vi "move_5.vi"(6 "Array 4":i32[](array[numeric]), 9 "Array 6":i32[](array[numeric]), 10 "Array in":i32[](array[numeric]), 11 "Enum in":enum16{"move4", "move4_1", "move4_2"}(ring)) -> (1 "Array 3":i32[](array[numeric]), 2 "Array out":i32[](array[numeric]), 3 "Enum out":T1(ring), 4 "Array 5":i32[](array[numeric]))   [LabVIEW 2016]
uses:
  <vilib>/NXT/Block Support/NXT_OutputPort.ctl
  <vilib>/NXT/NXTIO Xnodes/NXTIONodeSubVIs/NXTStopMotors.vi
  <vilib>/NXT/NXTIO Xnodes/NXTIONodeSubVIs/NXTMotorRunDistance.vi
  <vilib>/NXT/NXTIO Xnodes/NXTIONodeSubVIs/LEGOMotorStatus.vi
  <vilib>/NXT/NXTIO Xnodes/NXTIONodeSubVIs/NXTMoveMotors.vi
  <vilib>/NXT/NXTIO Xnodes/NXTIONodeSubVIs/LEGOResetMotors.vi
  <vilib>/NXT/Subs/LVHSConnector.ctl
  <vilib>/NXT/NXTIO Xnodes/AddressXNode/NXTIOAddress.xnode
  <vilib>/NXT/NXTIO Xnodes/NXTIOXNode/NXTIO.xnode
  <vilib>/NXT/LegoClasses/BrickReference/BrickReference.lvclass
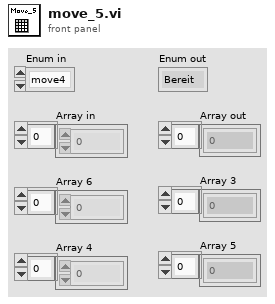
[diagram p1: front panel]
types:
  T1 = enum16{"Bereit", "Move 1", "Reference_pos", "Wait", "row1_check", "row2_check", "row3_check", "return", "move2", "move3", "move4", "move5", "end"}
  T2 = enum16{"forward", "right", "mark", "pause", "up", "return", "end"}
  T3 = typedef "NXT_OutputPort.ctl" = u8
  T4 = cluster{"Output Port":T3, "Output Port 2":T3, "Output Port 3":T3}
  T5 = enum16{"forward", "mark", "pause", "up", "return", "end"}
  T6 = typedef "LVHSConnector.ctl" = refnum<class "BrickReference.lvclass">
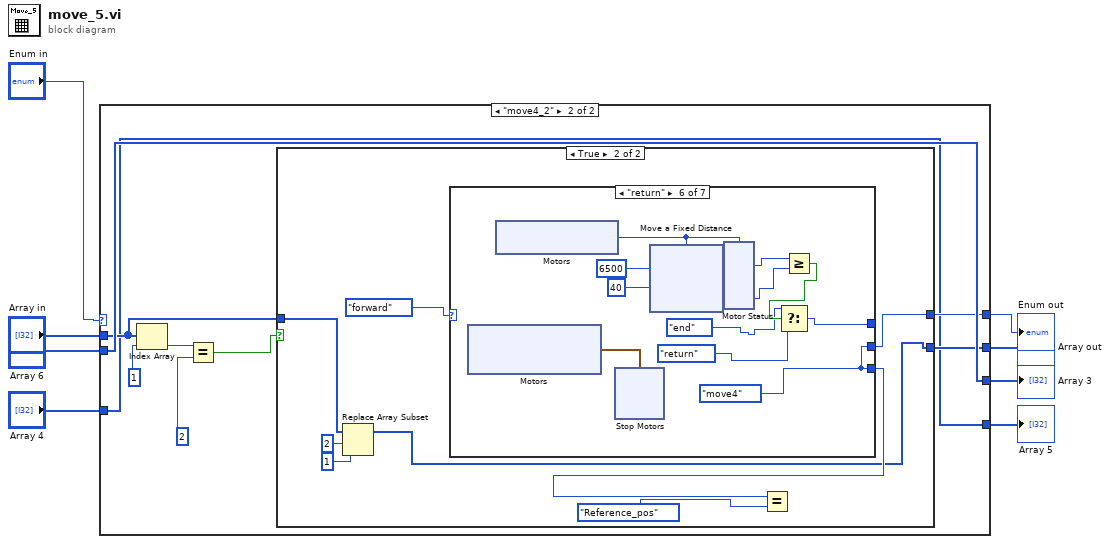
[diagram p0: block diagram]
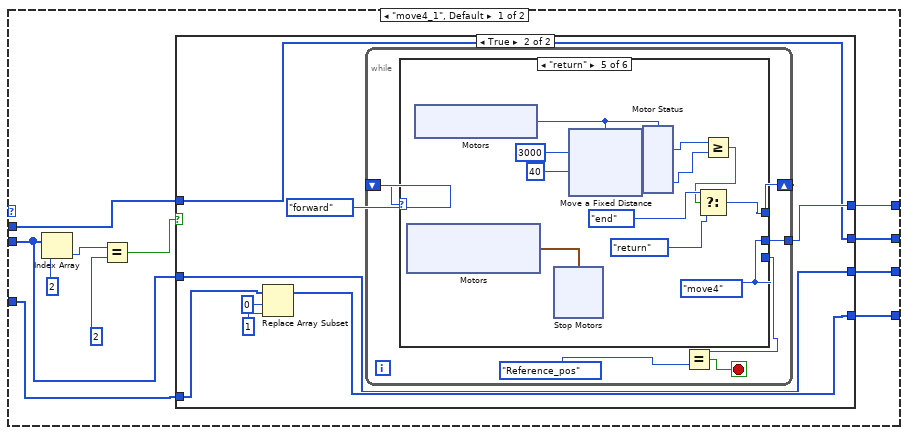
[diagram p2: hidden frame]
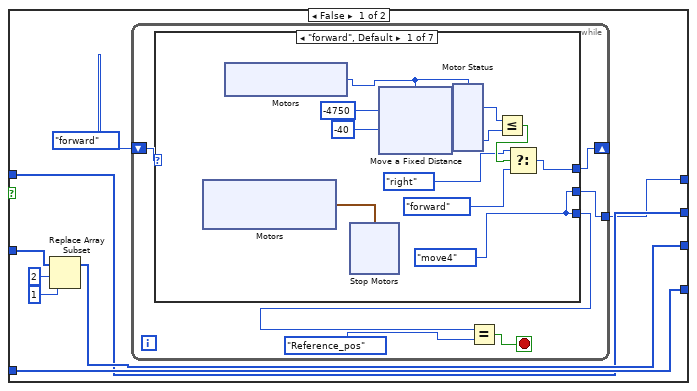
[diagram p3: hidden frame]
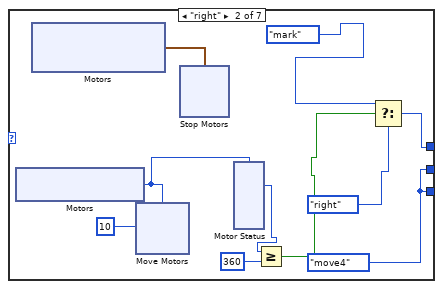
[diagram p4: hidden frame]
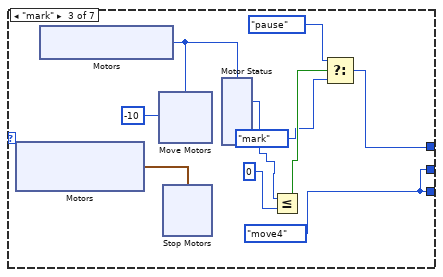
[diagram p5: hidden frame]
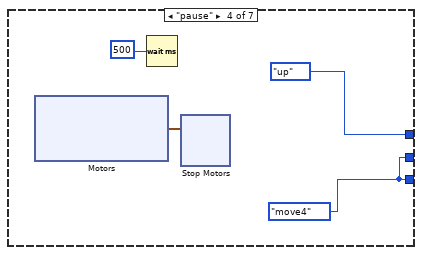
[diagram p6: hidden frame]
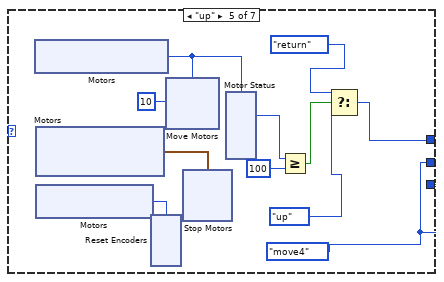
[diagram p7: hidden frame]
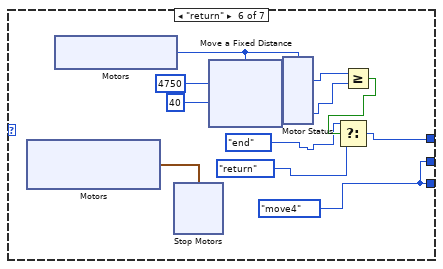
[diagram p8: hidden frame]
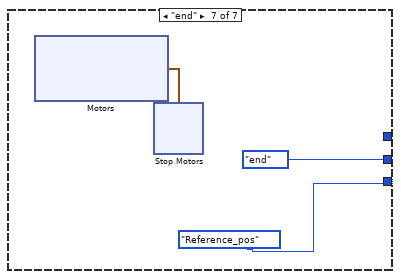
[diagram p9: hidden frame]
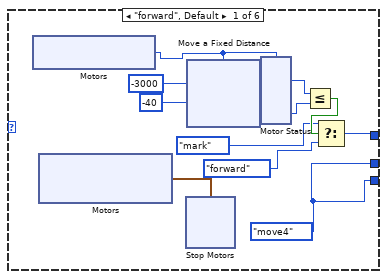
[diagram p10: hidden frame]
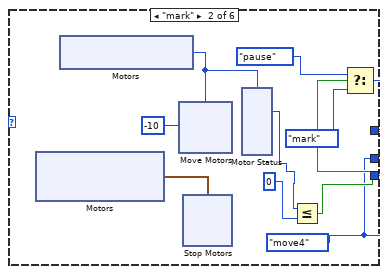
[diagram p11: hidden frame]
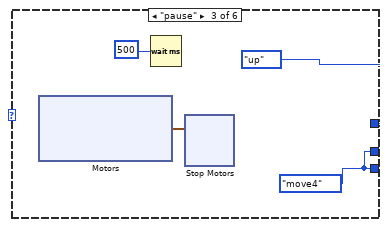
[diagram p12: hidden frame]
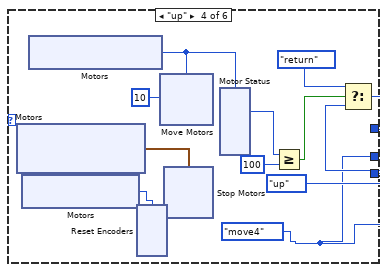
[diagram p13: hidden frame]
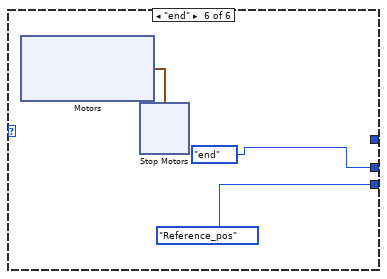
[diagram p14: hidden frame]
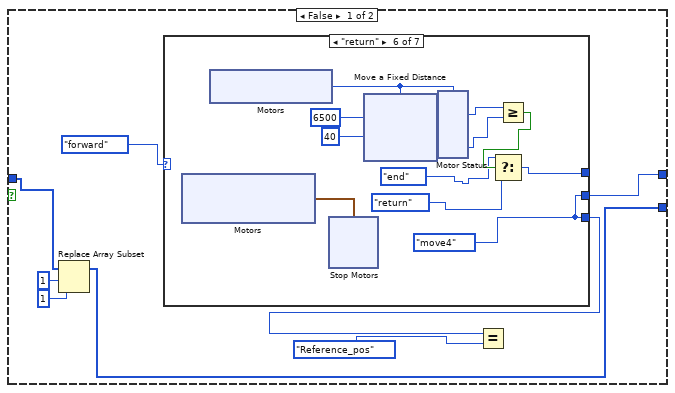
[diagram p15: hidden frame]
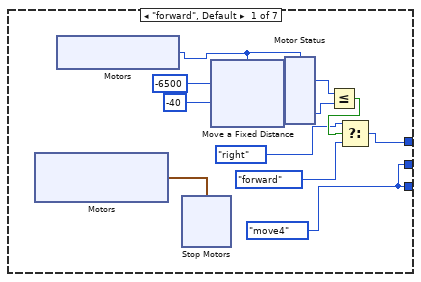
[diagram p16: hidden frame]
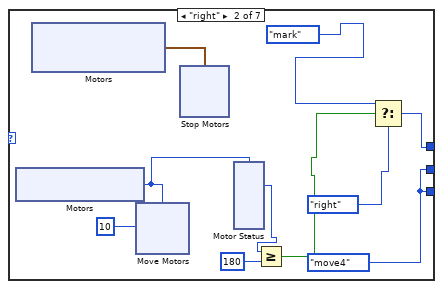
[diagram p17: hidden frame]
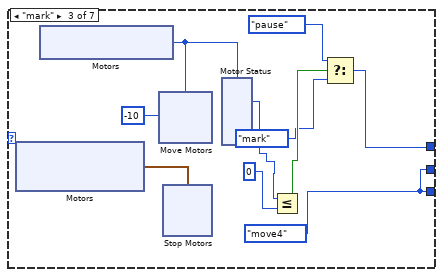
[diagram p18: hidden frame]
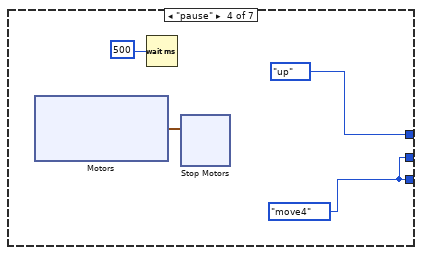
[diagram p19: hidden frame]
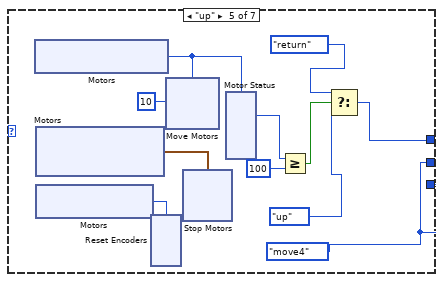
[diagram p20: hidden frame]
diagram:
  n1 = case shown="\"move4_2\"" "Enum in" {
    tunnel: "Array 6" -> [w13 w406]
    tunnel: [w15 w402] -> w2
    tunnel: "Array 4" -> [w14 w402]
    tunnel: [w12 w406] -> w4
    tunnel: [w11 w404] -> w5
    tunnel: "Array in" -> [w10 w405]
    tunnel: [w9 w403] -> w7
    frame "move4_1", Default {
      n2 = Index Array(array=w13, index=2) -> (element=w16:i32)
      n3 = Equal?(x=w16, y=2 ("element")) -> (x = y?=w18:bool)
      n4 = case shown="True" w18 {
        tunnel: [w24 w230] -> w15
        tunnel: w14 -> [w24 w231]
        tunnel: w13 -> [w23 w228]
        tunnel: [w22 w228] -> w12
        tunnel: [w21 w227] -> w11
        tunnel: w10 -> [w21 w227]
        tunnel: [w20 w229] -> w9
        frame False {
          n5 = Replace Array Subset(array=w23, new element=1 ("new element/subarray"), index=2) -> (w22:i32[])
          n6 = while {
            shift-right: [w29] -> _
            shift-left: T2."forward" -> [w30]
            tunnel: [w28] -> w20
            stop <- w32 stop-if-true
            n7 = case shown="\"forward\", Default" w30 {
              tunnel: [w34 w71 w103 T2."up" w146 w182 _] -> w29
              tunnel: [w43 w70 w102 w134 w145 w191 T1."Reference_pos"] -> w33
              tunnel: [w43 w70 w102 w134 w145 w191 T1."end"] -> w28
              frame "forward", Default {
                w39 = -4750 ("Distance 1")
                w43 = T1."move4"
                n8 = xnode "Motors"() -> ("Motor"=w44:cluster{"Port":T3, "Port":T3})
                n9 = xnode "Motors"() -> ("Motor"=w38:T3)
                n10 = xnode "Stop Motors"("Motors"=w44) -> ()  [unwired: 1 in, 1 out]
                n11 = xnode "Move a Fixed Distance"("Speed 1"=i8 -40, "Distance 1"=w39, "Motors"=w38) -> ("NXT/EV3"=w40:T6)  [unwired: 1 in]
                n12 = xnode "Motor Status"("Motors"=w38, "NXT/EV3"=w40) -> ("Position 1"=w41:i32)  [unwired: 2 out]
                n13 = Less Or Equal?(x=w41, y=w39) -> (x <= y?=w37:bool)
                n14 = Select(t=T2."right", s=w37, f=T2."forward") -> (s? t:f=w34:T2)
              }
              frame "right" {
                w70 = T1."move4"
                n15 = xnode "Motors"() -> ("Motor"=w79:T3)
                n16 = xnode "Motors"() -> ("Motor"=w78:cluster{"Port":T3, "Port":T3})
                n17 = xnode "Move Motors"("Power/Speed 1"=i8 10, "Motors"=w79) -> ()  [unwired: 1 in, 1 out]
                n18 = xnode "Stop Motors"("Motors"=w78) -> ()  [unwired: 1 in, 1 out]
                n19 = xnode "Motor Status"("Motors"=w79) -> ("Position 1"=w76:i32)  [unwired: 1 in, 2 out]
                n20 = Greater Or Equal?(x=w76, y=360) -> (x >= y?=w75:bool)
                n21 = Select(t=T2."mark", s=w75, f=T2."right") -> (s? t:f=w71:T2)
              }
              frame "mark" {
                w102 = T1."move4"
                n22 = xnode "Motors"() -> ("Motor"=w111:cluster{"Port":T3, "Port":T3})
                n23 = xnode "Motors"() -> ("Motor"=w109:T3)
                n24 = xnode "Move Motors"("Power/Speed 1"=i8 -10, "Motors"=w109) -> ()  [unwired: 1 in, 1 out]
                n25 = xnode "Stop Motors"("Motors"=w111) -> ()  [unwired: 1 in, 1 out]
                n26 = xnode "Motor Status"("Motors"=w109) -> ("Position 1"=w108:i32)  [unwired: 1 in, 2 out]
                n27 = Less Or Equal?(x=w108, y=0) -> (x <= y?=w106:bool)
                n28 = Select(t=T2."pause", s=w106, f=T2."mark") -> (s? t:f=w103:T2)
              }
              frame "pause" {
                w134 = T1."move4"
                n29 = xnode "Motors"() -> ("Motor"=w137:cluster{"Port":T3, "Port":T3, "Port":T3})
                n30 = Wait (ms)(milliseconds to wait=u32 500 ("millisecond timer value")) -> ()  [unwired: 1 out]
                n31 = xnode "Stop Motors"("Motors"=w137) -> ()  [unwired: 1 in, 1 out]
              }
              frame "up" {
                w145 = T1."move4"
                n32 = xnode "Motors"() -> ("Motor"=w150:T3)
                n33 = xnode "Motors"() -> ("Motor"=w153:cluster{"Port":T3, "Port":T3})
                n34 = xnode "Motors"() -> ("Motor"=w144:T3)
                n35 = xnode "Reset Encoders"("Motors"=w144) -> ()  [unwired: 1 in, 1 out]
                n36 = xnode "Move Motors"("Power/Speed 1"=i8 10, "Motors"=w150) -> ()  [unwired: 1 in, 1 out]
                n37 = xnode "Stop Motors"("Motors"=w153) -> ()  [unwired: 1 in, 1 out]
                n38 = xnode "Motor Status"("Motors"=w150) -> ("Position 1"=w151:i32)  [unwired: 1 in, 2 out]
                n39 = Greater Or Equal?(x=w151, y=100) -> (x >= y?=w152:bool)
                n40 = Select(t=T2."return", s=w152, f=T2."up") -> (s? t:f=w146:T2)
              }
              frame "return" {
                w186 = 4750 ("Distance 1")
                w191 = T1."move4"
                n41 = xnode "Motors"() -> ("Motor"=w192:cluster{"Port":T3, "Port":T3})
                n42 = xnode "Motors"() -> ("Motor"=w189:T3)
                n43 = xnode "Stop Motors"("Motors"=w192) -> ()  [unwired: 1 in, 1 out]
                n44 = xnode "Move a Fixed Distance"("Speed 1"=i8 40, "Distance 1"=w186, "Motors"=w189) -> ("NXT/EV3"=w188:T6)  [unwired: 1 in]
                n45 = xnode "Motor Status"("Motors"=w189, "NXT/EV3"=w188) -> ("Position 1"=w187:i32)  [unwired: 2 out]
                n46 = Greater Or Equal?(x=w187, y=w186) -> (x >= y?=w185:bool)
                n47 = Select(t=T2."end", s=w185, f=T2."return") -> (s? t:f=w182:T2)
              }
              frame "end" {
                n48 = xnode "Motors"() -> ("Motor"=w219:cluster{"Port":T3, "Port":T3, "Port":T3})
                n49 = xnode "Stop Motors"("Motors"=w219) -> ()  [unwired: 1 in, 1 out]
              }
            }
            n50 = Equal?(x=w33, y=T1."Reference_pos") -> (x = y?=w32:bool)
          }
        }
        frame True {
          n51 = Replace Array Subset(array=w231, new element=1 ("new element/subarray"), index=0) -> (w230:i32[])
          n52 = while {
            shift-right: [w240] -> _
            shift-left: T5."forward" -> [w239]
            tunnel: [w235] -> w229
            stop <- w237 stop-if-true
            n53 = case shown="\"return\"" w239 {
              tunnel: [w241 w284 T5."up" w326 w358 _] -> w240
              tunnel: [w250 w277 w309 w320 w366 T1."Reference_pos"] -> w238
              tunnel: [w250 w277 w309 w320 w366 T1."end"] -> w235
              frame "forward", Default {
                w246 = -3000 ("Distance 1")
                w250 = T1."move4"
                n54 = xnode "Motors"() -> ("Motor"=w245:T3)
                n55 = xnode "Motors"() -> ("Motor"=w251:cluster{"Port":T3, "Port":T3})
                n56 = xnode "Stop Motors"("Motors"=w251) -> ()  [unwired: 1 in, 1 out]
                n57 = xnode "Move a Fixed Distance"("Speed 1"=i8 -40, "Distance 1"=w246, "Motors"=w245) -> ("NXT/EV3"=w247:T6)  [unwired: 1 in]
                n58 = xnode "Motor Status"("Motors"=w245, "NXT/EV3"=w247) -> ("Position 1"=w248:i32)  [unwired: 2 out]
                n59 = Less Or Equal?(x=w248, y=w246) -> (x <= y?=w244:bool)
                n60 = Select(t=T5."mark", s=w244, f=T5."forward") -> (s? t:f=w241:T5)
              }
              frame "mark" {
                w277 = T1."move4"
                n61 = xnode "Motors"() -> ("Motor"=w286:cluster{"Port":T3, "Port":T3})
                n62 = xnode "Motors"() -> ("Motor"=w281:T3)
                n63 = xnode "Move Motors"("Power/Speed 1"=i8 -10, "Motors"=w281) -> ()  [unwired: 1 in, 1 out]
                n64 = xnode "Stop Motors"("Motors"=w286) -> ()  [unwired: 1 in, 1 out]
                n65 = xnode "Motor Status"("Motors"=w281) -> ("Position 1"=w280:i32)  [unwired: 1 in, 2 out]
                n66 = Less Or Equal?(x=w280, y=0) -> (x <= y?=w278:bool)
                n67 = Select(t=T5."pause", s=w278, f=T5."mark") -> (s? t:f=w284:T5)
              }
              frame "pause" {
                w309 = T1."move4"
                n68 = xnode "Motors"() -> ("Motor"=w312:cluster{"Port":T3, "Port":T3, "Port":T3})
                n69 = Wait (ms)(milliseconds to wait=u32 500 ("millisecond timer value")) -> ()  [unwired: 1 out]
                n70 = xnode "Stop Motors"("Motors"=w312) -> ()  [unwired: 1 in, 1 out]
              }
              frame "up" {
                w320 = T1."move4"
                n71 = xnode "Motors"() -> ("Motor"=w328:cluster{"Port":T3, "Port":T3})
                n72 = xnode "Motors"() -> ("Motor"=w319:T3)
                n73 = xnode "Motors"() -> ("Motor"=w322:T3)
                n74 = xnode "Reset Encoders"("Motors"=w319) -> ()  [unwired: 1 in, 1 out]
                n75 = xnode "Move Motors"("Power/Speed 1"=i8 10, "Motors"=w322) -> ()  [unwired: 1 in, 1 out]
                n76 = xnode "Stop Motors"("Motors"=w328) -> ()  [unwired: 1 in, 1 out]
                n77 = xnode "Motor Status"("Motors"=w322) -> ("Position 1"=w323:i32)  [unwired: 1 in, 2 out]
                n78 = Greater Or Equal?(x=w323, y=100) -> (x >= y?=w327:bool)
                n79 = Select(t=T5."return", s=w327, f=T5."up") -> (s? t:f=w326:T5)
              }
              frame "return" {
                w361 = 3000 ("Distance 1")
                w366 = T1."move4"
                n80 = xnode "Motors"() -> ("Motor"=w367:cluster{"Port":T3, "Port":T3})
                n81 = xnode "Motors"() -> ("Motor"=w364:T3)
                n82 = xnode "Stop Motors"("Motors"=w367) -> ()  [unwired: 1 in, 1 out]
                n83 = xnode "Move a Fixed Distance"("Speed 1"=i8 40, "Distance 1"=w361, "Motors"=w364) -> ("NXT/EV3"=w363:T6)  [unwired: 1 in]
                n84 = xnode "Motor Status"("Motors"=w364, "NXT/EV3"=w363) -> ("Position 1"=w362:i32)  [unwired: 2 out]
                n85 = Greater Or Equal?(x=w362, y=w361) -> (x >= y?=w357:bool)
                n86 = Select(t=T5."end", s=w357, f=T5."return") -> (s? t:f=w358:T5)
              }
              frame "end" {
                n87 = xnode "Motors"() -> ("Motor"=w395:cluster{"Port":T3, "Port":T3, "Port":T3})
                n88 = xnode "Stop Motors"("Motors"=w395) -> ()  [unwired: 1 in, 1 out]
              }
            }
            n89 = Equal?(x=w238, y=T1."Reference_pos") -> (x = y?=w237:bool)
          }
        }
      }
    }
    frame "move4_2" {
      n90 = Index Array(array=w405, index=1) -> (element=w407:i32)
      n91 = Equal?(x=w407, y=2 ("element")) -> (x = y?=w409:bool)
      n92 = case shown="True" w409 {
        tunnel: w405 -> [w413 w614]
        tunnel: [w412 w613] -> w404
        tunnel: [w411 w612] -> w403
        frame False {
          n93 = Replace Array Subset(array=w413, new element=1 ("new element/subarray"), index=1) -> (w412:i32[])
          n94 = case shown="\"return\"" T2."forward" {
            tunnel: [w419 w456 w488 T2."up" w531 w567 _] -> _
            tunnel: [w428 w455 w487 w519 w530 w576 T1."Reference_pos"] -> w416
            tunnel: [w428 w455 w487 w519 w530 w576 T1."end"] -> w411
            frame "forward", Default {
              w424 = -6500 ("Distance 1")
              w428 = T1."move4"
              n95 = xnode "Motors"() -> ("Motor"=w429:cluster{"Port":T3, "Port":T3})
              n96 = xnode "Motors"() -> ("Motor"=w423:T3)
              n97 = xnode "Stop Motors"("Motors"=w429) -> ()  [unwired: 1 in, 1 out]
              n98 = xnode "Move a Fixed Distance"("Speed 1"=i8 -40, "Distance 1"=w424, "Motors"=w423) -> ("NXT/EV3"=w425:T6)  [unwired: 1 in]
              n99 = xnode "Motor Status"("Motors"=w423, "NXT/EV3"=w425) -> ("Position 1"=w426:i32)  [unwired: 2 out]
              n100 = Less Or Equal?(x=w426, y=w424) -> (x <= y?=w422:bool)
              n101 = Select(t=T2."right", s=w422, f=T2."forward") -> (s? t:f=w419:T2)
            }
            frame "right" {
              w455 = T1."move4"
              n102 = xnode "Motors"() -> ("Motor"=w464:T3)
              n103 = xnode "Motors"() -> ("Motor"=w463:cluster{"Port":T3, "Port":T3})
              n104 = xnode "Move Motors"("Power/Speed 1"=i8 10, "Motors"=w464) -> ()  [unwired: 1 in, 1 out]
              n105 = xnode "Stop Motors"("Motors"=w463) -> ()  [unwired: 1 in, 1 out]
              n106 = xnode "Motor Status"("Motors"=w464) -> ("Position 1"=w461:i32)  [unwired: 1 in, 2 out]
              n107 = Greater Or Equal?(x=w461, y=180) -> (x >= y?=w460:bool)
              n108 = Select(t=T2."mark", s=w460, f=T2."right") -> (s? t:f=w456:T2)
            }
            frame "mark" {
              w487 = T1."move4"
              n109 = xnode "Motors"() -> ("Motor"=w496:cluster{"Port":T3, "Port":T3})
              n110 = xnode "Motors"() -> ("Motor"=w494:T3)
              n111 = xnode "Move Motors"("Power/Speed 1"=i8 -10, "Motors"=w494) -> ()  [unwired: 1 in, 1 out]
              n112 = xnode "Stop Motors"("Motors"=w496) -> ()  [unwired: 1 in, 1 out]
              n113 = xnode "Motor Status"("Motors"=w494) -> ("Position 1"=w493:i32)  [unwired: 1 in, 2 out]
              n114 = Less Or Equal?(x=w493, y=0) -> (x <= y?=w491:bool)
              n115 = Select(t=T2."pause", s=w491, f=T2."mark") -> (s? t:f=w488:T2)
            }
            frame "pause" {
              w519 = T1."move4"
              n116 = xnode "Motors"() -> ("Motor"=w522:cluster{"Port":T3, "Port":T3, "Port":T3})
              n117 = Wait (ms)(milliseconds to wait=u32 500 ("millisecond timer value")) -> ()  [unwired: 1 out]
              n118 = xnode "Stop Motors"("Motors"=w522) -> ()  [unwired: 1 in, 1 out]
            }
            frame "up" {
              w530 = T1."move4"
              n119 = xnode "Motors"() -> ("Motor"=w535:T3)
              n120 = xnode "Motors"() -> ("Motor"=w538:cluster{"Port":T3, "Port":T3})
              n121 = xnode "Motors"() -> ("Motor"=w529:T3)
              n122 = xnode "Reset Encoders"("Motors"=w529) -> ()  [unwired: 1 in, 1 out]
              n123 = xnode "Move Motors"("Power/Speed 1"=i8 10, "Motors"=w535) -> ()  [unwired: 1 in, 1 out]
              n124 = xnode "Stop Motors"("Motors"=w538) -> ()  [unwired: 1 in, 1 out]
              n125 = xnode "Motor Status"("Motors"=w535) -> ("Position 1"=w536:i32)  [unwired: 1 in, 2 out]
              n126 = Greater Or Equal?(x=w536, y=100) -> (x >= y?=w537:bool)
              n127 = Select(t=T2."return", s=w537, f=T2."up") -> (s? t:f=w531:T2)
            }
            frame "return" {
              w571 = 6500 ("Distance 1")
              w576 = T1."move4"
              n128 = xnode "Motors"() -> ("Motor"=w577:cluster{"Port":T3, "Port":T3})
              n129 = xnode "Motors"() -> ("Motor"=w574:T3)
              n130 = xnode "Stop Motors"("Motors"=w577) -> ()  [unwired: 1 in, 1 out]
              n131 = xnode "Move a Fixed Distance"("Speed 1"=i8 40, "Distance 1"=w571, "Motors"=w574) -> ("NXT/EV3"=w573:T6)  [unwired: 1 in]
              n132 = xnode "Motor Status"("Motors"=w574, "NXT/EV3"=w573) -> ("Position 1"=w572:i32)  [unwired: 2 out]
              n133 = Greater Or Equal?(x=w572, y=w571) -> (x >= y?=w570:bool)
              n134 = Select(t=T2."end", s=w570, f=T2."return") -> (s? t:f=w567:T2)
            }
            frame "end" {
              n135 = xnode "Motors"() -> ("Motor"=w604:cluster{"Port":T3, "Port":T3, "Port":T3})
              n136 = xnode "Stop Motors"("Motors"=w604) -> ()  [unwired: 1 in, 1 out]
            }
          }
          n137 = Equal?(x=w416, y=T1."Reference_pos") -> ()  [unwired: 1 out]
        }
        frame True {
          n138 = Replace Array Subset(array=w614, new element=1 ("new element/subarray"), index=2) -> (w613:i32[])
          n139 = case shown="\"return\"" T2."forward" {
            tunnel: [w620 w657 w689 T2."up" w732 w768 _] -> _
            tunnel: [w629 w656 w688 w720 w731 w777 T1."Reference_pos"] -> w617
            tunnel: [w629 w656 w688 w720 w731 w777 T1."end"] -> w612
            frame "forward", Default {
              w625 = -6500 ("Distance 1")
              w629 = T1."move4"
              n140 = xnode "Motors"() -> ("Motor"=w630:cluster{"Port":T3, "Port":T3})
              n141 = xnode "Motors"() -> ("Motor"=w624:T3)
              n142 = xnode "Stop Motors"("Motors"=w630) -> ()  [unwired: 1 in, 1 out]
              n143 = xnode "Move a Fixed Distance"("Speed 1"=i8 -40, "Distance 1"=w625, "Motors"=w624) -> ("NXT/EV3"=w626:T6)  [unwired: 1 in]
              n144 = xnode "Motor Status"("Motors"=w624, "NXT/EV3"=w626) -> ("Position 1"=w627:i32)  [unwired: 2 out]
              n145 = Less Or Equal?(x=w627, y=w625) -> (x <= y?=w623:bool)
              n146 = Select(t=T2."right", s=w623, f=T2."forward") -> (s? t:f=w620:T2)
            }
            frame "right" {
              w656 = T1."move4"
              n147 = xnode "Motors"() -> ("Motor"=w665:T3)
              n148 = xnode "Motors"() -> ("Motor"=w664:cluster{"Port":T3, "Port":T3})
              n149 = xnode "Move Motors"("Power/Speed 1"=i8 10, "Motors"=w665) -> ()  [unwired: 1 in, 1 out]
              n150 = xnode "Stop Motors"("Motors"=w664) -> ()  [unwired: 1 in, 1 out]
              n151 = xnode "Motor Status"("Motors"=w665) -> ("Position 1"=w662:i32)  [unwired: 1 in, 2 out]
              n152 = Greater Or Equal?(x=w662, y=360) -> (x >= y?=w661:bool)
              n153 = Select(t=T2."mark", s=w661, f=T2."right") -> (s? t:f=w657:T2)
            }
            frame "mark" {
              w688 = T1."move4"
              n154 = xnode "Motors"() -> ("Motor"=w697:cluster{"Port":T3, "Port":T3})
              n155 = xnode "Motors"() -> ("Motor"=w695:T3)
              n156 = xnode "Move Motors"("Power/Speed 1"=i8 -10, "Motors"=w695) -> ()  [unwired: 1 in, 1 out]
              n157 = xnode "Stop Motors"("Motors"=w697) -> ()  [unwired: 1 in, 1 out]
              n158 = xnode "Motor Status"("Motors"=w695) -> ("Position 1"=w694:i32)  [unwired: 1 in, 2 out]
              n159 = Less Or Equal?(x=w694, y=0) -> (x <= y?=w692:bool)
              n160 = Select(t=T2."pause", s=w692, f=T2."mark") -> (s? t:f=w689:T2)
            }
            frame "pause" {
              w720 = T1."move4"
              n161 = xnode "Motors"() -> ("Motor"=w723:cluster{"Port":T3, "Port":T3, "Port":T3})
              n162 = Wait (ms)(milliseconds to wait=u32 500 ("millisecond timer value")) -> ()  [unwired: 1 out]
              n163 = xnode "Stop Motors"("Motors"=w723) -> ()  [unwired: 1 in, 1 out]
            }
            frame "up" {
              w731 = T1."move4"
              n164 = xnode "Motors"() -> ("Motor"=w736:T3)
              n165 = xnode "Motors"() -> ("Motor"=w739:cluster{"Port":T3, "Port":T3})
              n166 = xnode "Motors"() -> ("Motor"=w730:T3)
              n167 = xnode "Reset Encoders"("Motors"=w730) -> ()  [unwired: 1 in, 1 out]
              n168 = xnode "Move Motors"("Power/Speed 1"=i8 10, "Motors"=w736) -> ()  [unwired: 1 in, 1 out]
              n169 = xnode "Stop Motors"("Motors"=w739) -> ()  [unwired: 1 in, 1 out]
              n170 = xnode "Motor Status"("Motors"=w736) -> ("Position 1"=w737:i32)  [unwired: 1 in, 2 out]
              n171 = Greater Or Equal?(x=w737, y=100) -> (x >= y?=w738:bool)
              n172 = Select(t=T2."return", s=w738, f=T2."up") -> (s? t:f=w732:T2)
            }
            frame "return" {
              w772 = 6500 ("Distance 1")
              w777 = T1."move4"
              n173 = xnode "Motors"() -> ("Motor"=w778:cluster{"Port":T3, "Port":T3})
              n174 = xnode "Motors"() -> ("Motor"=w775:T3)
              n175 = xnode "Stop Motors"("Motors"=w778) -> ()  [unwired: 1 in, 1 out]
              n176 = xnode "Move a Fixed Distance"("Speed 1"=i8 40, "Distance 1"=w772, "Motors"=w775) -> ("NXT/EV3"=w774:T6)  [unwired: 1 in]
              n177 = xnode "Motor Status"("Motors"=w775, "NXT/EV3"=w774) -> ("Position 1"=w773:i32)  [unwired: 2 out]
              n178 = Greater Or Equal?(x=w773, y=w772) -> (x >= y?=w771:bool)
              n179 = Select(t=T2."end", s=w771, f=T2."return") -> (s? t:f=w768:T2)
            }
            frame "end" {
              n180 = xnode "Motors"() -> ("Motor"=w805:cluster{"Port":T3, "Port":T3, "Port":T3})
              n181 = xnode "Stop Motors"("Motors"=w805) -> ()  [unwired: 1 in, 1 out]
            }
          }
          n182 = Equal?(x=w617, y=T1."Reference_pos") -> ()  [unwired: 1 out]
        }
      }
    }
  }
  "Enum out" <- w7
  "Array out" <- w5
  "Array 3" <- w4
  "Array 5" <- w2
